vi "kw_hamming.vi"(11 "L Hamming":i32) -> (3 "Kw Hamming":dbl)   [LabVIEW 2020]
uses:
  <vilib>/Analysis/4window.llb/Hamming Window (DBL).vi
  <vilib>/Analysis/4window.llb/AllCosWindow (DBL).vi
  <vilib>/Analysis/NI_AALPro.lvlib
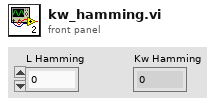
[diagram p1: front panel]
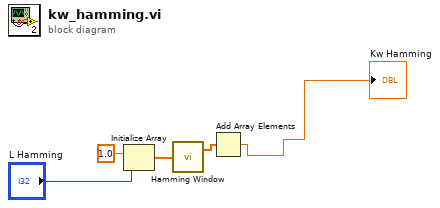
[diagram p0: block diagram]
diagram:
  n1 = Initialize Array(1.0 ("element"), "L Hamming") -> (w3:dbl[])
  n2 = call-poly <vilib>:"Hamming Window.vi"("X"=w3) -> ("Windowed X"=w4:dbl[])  [unwired: 1 out]
  n3 = Add Array Elements(numeric array=w4) -> (sum=→"Kw Hamming":dbl)
